vi "Poisson Random.vi"(6 "seed":i32=-1, 7 "reset":bool, 10 "lambda":dbl=1.0, 11 "samples":i32=128) -> (0 "error":i32, 3 "Poisson random data":i32[](array[numeric]))   [LabVIEW 2014, in "NI_Gmath.lvlib"]
doc: "Generates random values from a variate X, where X describes the selected distribution type. You must manually select the polymorphic instance to use."
uses:
  NI_Gmath.lvlib
  st_error_code.ctl
  NI_AALBase.lvlib
panel:
  # "Poisson Random"
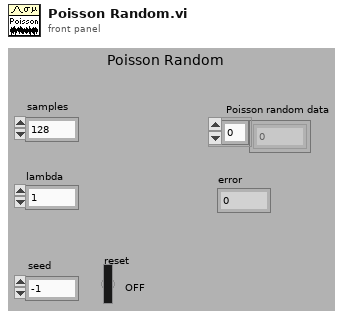
[diagram p1: front panel]
types:
  T1 = typedef "NI_Gmath.lvlib/st_error_code.ctl" = i32
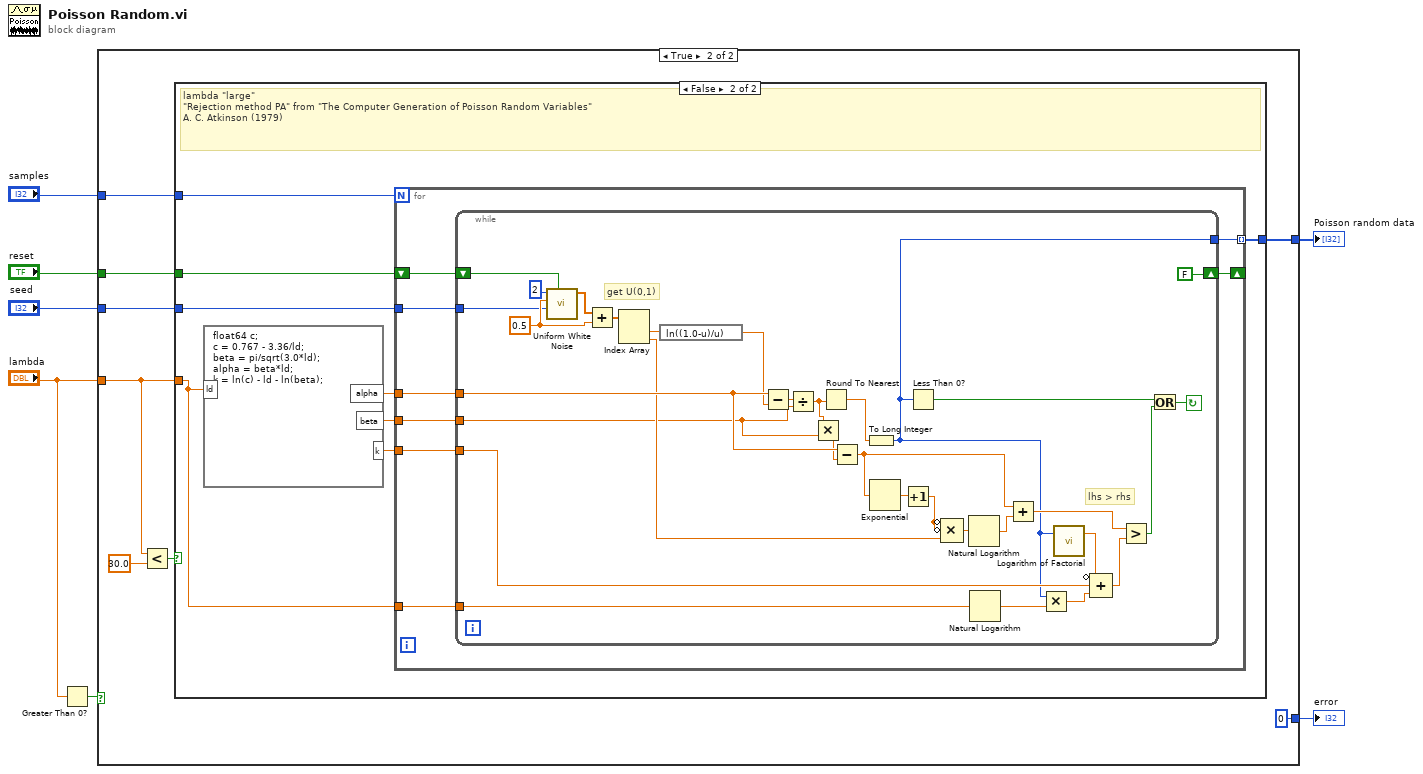
[diagram p0: block diagram]
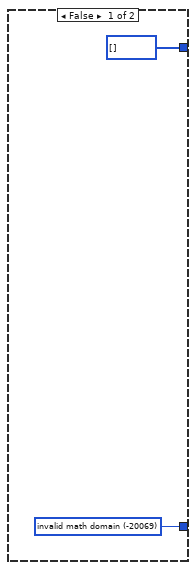
[diagram p2: hidden frame]
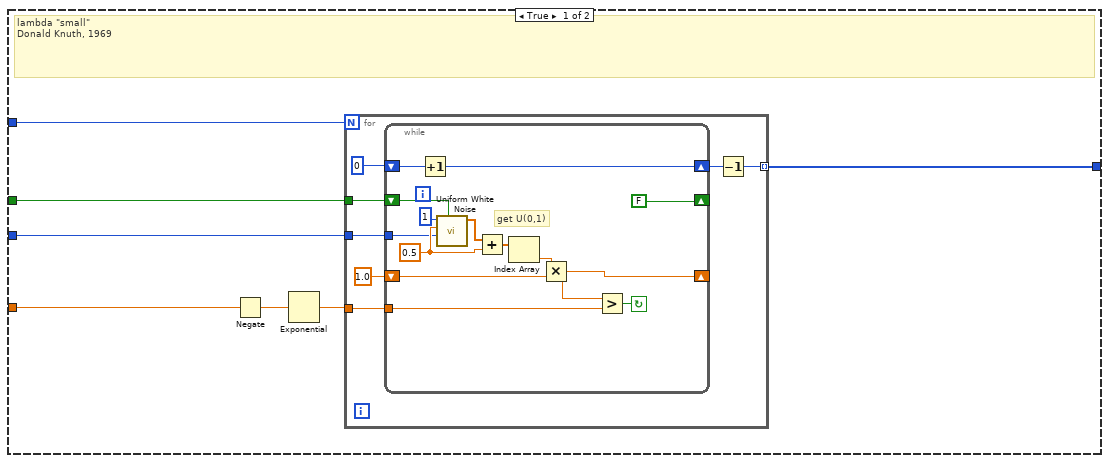
[diagram p3: hidden frame]
diagram:
  n1 = Greater Than 0?(x="lambda") -> (x > 0?=w7:bool)
  n2 = case shown="True" w7 {
    tunnel: [i32[] [] w16] -> w2
    tunnel: "lambda" -> [_ w10]
    tunnel: [w8 0 ("invalid math domain")] -> w1
    tunnel: "reset" -> [_ w15]
    tunnel: "samples" -> [_ w14]
    tunnel: "seed" -> [_ w13]
    frame False {
      w8 = T1 -20069 items=["invalid math domain"=-20069, "Fourier interpolation size m >= n"=-20070, "empty array"=-20003] ("stat interp error code")
    }
    frame True {
      n3 = Less?(x=w10, y=30.0) -> (x < y?=w12:bool)
      n4 = case shown="False" w12 {
        tunnel: w10 -> [w24 w47]
        tunnel: [w21 w46] -> w16
        tunnel: w15 -> [w20 w53]
        tunnel: w14 -> [w19 w52]
        tunnel: w13 -> [w18 w51]
        frame True {
          # "lambda \"small\"\nDonald Knuth, 1969"
          n5 = Negate(x=w24) -> (-x=w23:dbl)
          n6 = Exponential(1:w23) -> (0:w22:dbl)
          n7 = for {
            N: w19 -> [_]
            tunnel: w22 -> [w30]
            tunnel: [w28] -> w21 mode=indexing
            tunnel: w20 -> [w27]
            tunnel: w18 -> [w26]
            n8 = while {
              shift-right: [w44] -> w29
              shift-left: 0 -> [w45]
              shift-right: [FALSE ("reset")] -> _
              shift-left: w27 -> [w38]
              tunnel: w30 -> [w37]
              tunnel: w26 -> [w35]
              shift-right: [w32] -> _
              shift-left: 1.0 -> [w33]
              stop <- w36 continue-if-true
              w41 = 0.5 ("amplitude")
              # "get U(0,1)"
              n9 = Increment(x=w45) -> (x+1=w44:i32)
              n10 = call "Uniform White Noise.vi"("initialize?"=w38, "seed"=w35, "amplitude"=w41, "samples"=1) -> ("uniform white noise"=w42:dbl[])  [unwired: 6 in, 1 out]
              n11 = Add(x=w42, y=w41) -> (x+y=w43:dbl[])
              n12 = Index Array(array=w43) -> (element=w34:dbl)  [unwired: 1 in]
              n13 = Multiply(x=w34, y=w33) -> (x*y=w32:dbl)
              n14 = Greater?(x=w32, y=w37) -> (0:w36:bool)
            }
            n15 = Decrement(x=w29) -> (x-1=w28:i32)
          }
        }
        frame False {
          # "lambda \"large\"\n\"Rejection method PA\" from \"The Computer Generation of Poisson Random Variables\"\nA. C. Atkinson (1979)"
          n16 = formula code="float64 c;\nc = 0.767 - 3.36/ld;\nbeta = pi/sqrt(3.0*ld);\nalpha = beta*ld;\nk = ln(c) - ld - ln(beta);"("ld"=w47) -> ("k"=w48:dbl, "beta"=w49:dbl, "alpha"=w50:dbl)
          n17 = for {
            N: w52 -> [_]
            tunnel: w51 -> [w60]
            tunnel: w50 -> [w59]
            tunnel: w49 -> [w58]
            tunnel: w48 -> [w57]
            tunnel: w47 -> [w56]
            tunnel: [w55] -> w46 mode=indexing
            shift-right: [w54] -> _
            shift-left: w53 -> [w61]
            n18 = while {
              shift-right: [FALSE ("reset")] -> w54
              shift-left: w61 -> [w88]
              tunnel: w60 -> [w87]
              tunnel: w59 -> [w83]
              tunnel: w58 -> [w62]
              tunnel: w57 -> [w72]
              tunnel: w56 -> [w75]
              tunnel: [w66] -> w55
              stop <- w84 continue-if-true
              w91 = 0.5 ("amplitude")
              # "lhs > rhs"
              # "get U(0,1)"
              n19 = call "Uniform White Noise.vi"("initialize?"=w88, "seed"=w87, "amplitude"=w91, "samples"=2) -> ("uniform white noise"=w92:dbl[])  [unwired: 6 in, 1 out]
              n20 = Add(x=w92, y=w91) -> (x+y=w93:dbl[])
              n21 = Index Array(array=w93) -> (element #1=w86:dbl, element #2=w79:dbl)  [unwired: 2 in]
              n22 = expression code="ln((1.0-u)/u)"(w86) -> (w65:dbl)
              n23 = Subtract(x=w83, y=w65) -> (x-y=w64:dbl)
              n24 = Divide(x=w64, y=w62) -> (x/y=w63:dbl)
              n25 = Multiply(x=w63, y=w62) -> (x*y=w82:dbl)
              n26 = Round To Nearest(number=w63) -> (nearest integer value=w67:dbl)
              n27 = Subtract(x=w83, y=w82) -> (x-y=w77:dbl)
              n28 = To Long Integer(number=w67) -> (32bit integer=w66:i32)
              n29 = Exponential(1:w77) -> (0:w81:dbl)
              n30 = Increment(x=w81) -> (x+1=w80:dbl)
              n31 = Less Than 0?(x=w66) -> (x < 0?=w85:bool)
              n32 = Compound Arithmetic op=MULTIPLY(invert w80, invert w80, w79) -> (w78:dbl)
              n33 = Natural Logarithm(1:w78) -> (0:w76:dbl)
              n34 = Natural Logarithm(1:w75) -> (0:w74:dbl)
              n35 = Add(x=w77, y=w76) -> (x+y=w69:dbl)
              n36 = Multiply(x=w66, y=w74) -> (x*y=w73:dbl)
              n37 = call "Logarithm of Factorial.vi"("n"=w66) -> ("ln(n!)"=w71:dbl)  [unwired: 2 in]
              n38 = Compound Arithmetic op=ADD(invert w71, w72, w73) -> (w70:dbl)
              n39 = Greater?(x=w69, y=w70) -> (0:w68:bool)
              n40 = Or(x=w85, y=w68) -> (x .or. y?=w84:bool)
            }
          }
        }
      }
    }
  }
  "error" <- w1
  "Poisson random data" <- w2
